vi "Register Logger.vi"(8 "error in (no error)":errorcluster, 9 "Task ID":string, 10 "EnQr":refnum<class "Message Enqueuer.lvclass">, 11 "LoggingAPI in":refnum<class "LoggingAPI.lvclass">) -> (0 "error out":errorcluster, 3 "LoggingAPI out":refnum<class "LoggingAPI.lvclass">)   [LabVIEW 2020, in "VolatusData.lvlib" / "LoggingAPI.lvclass"]
uses:
  LoggingAPI.lvclass
  <vilib>/ActorFramework/Message Enqueuer/Message Enqueuer.lvclass
  LoggingAPI.lvclass/LoggingAPI.ctl
  LoggingManager Messages/Register Logger Msg/Register Logger Msg.lvclass/Register Logger Msg.ctl
  <vilib>/ActorFramework/Message Enqueuer/Message Enqueuer.lvclass/Message Enqueuer.ctl
  <vilib>/ActorFramework/Message Enqueuer/Enqueue.vi
  LoggingManager Messages/Register Logger Msg/Register Logger Msg.lvclass
  C:/Program Files (x86)/National Instruments/LabVIEW 2020/vi.lib/ActorFramework/Message/Message.lvclass
  <vilib>/ActorFramework/Message Priority Queue/Priority Enqueue.vi
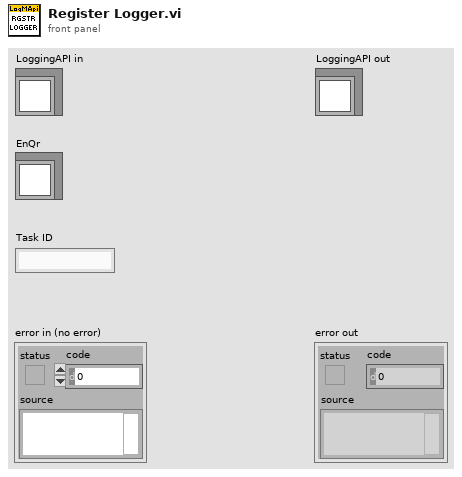
[diagram p1: front panel]
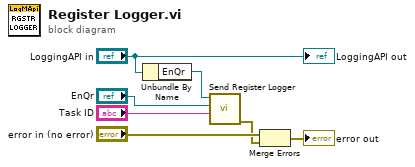
[diagram p0: block diagram]
diagram:
  n1 = Unbundle By Name("LoggingAPI in") -> ("EnQr"=w5:refnum<class "Message Enqueuer.lvclass">)
  n2 = call "Send Register Logger.vi"("Task ID"="Task ID", "EnQr"="EnQr", "Message Enqueuer"=w5) -> ("error out"=w1:errorcluster)  [unwired: 7 in, 1 out]
  n3 = Merge Errors("error in (no error)", w1) -> (→"error out":errorcluster)
  "LoggingAPI out" <- "LoggingAPI in"
